vi "Log Data.vi"(8 "error in (no error)":T1 caption="entrée d'erreur (pas d'erreur)", 10 "File d'attente de données":refnum<queue>, 11 "Configuration de l'enregistrement":T2) -> (0 "error out":T1 caption="sortie d'erreur")   [LabVIEW 2018, in "Logging.lvlib"]
doc: "Ce VI utilise la fonction TDMS - Écrire pour écrire des données dans un fichier TDMS."
uses:
  Logging.lvlib
  Logging Configuration.ctl
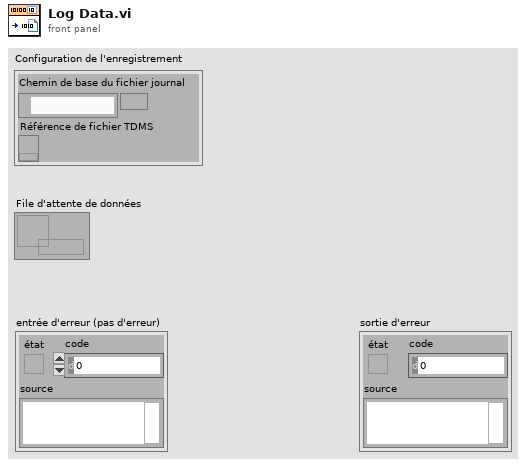
[diagram p1: front panel]
types:
  T1 = cluster{"état":bool, "code":i32, "source":string}
  T2 = typedef "Logging.lvlib/Logging Configuration.ctl" = cluster{"Chemin de base du fichier journal":path, "Référence de fichier TDMS":refnum<k34>}
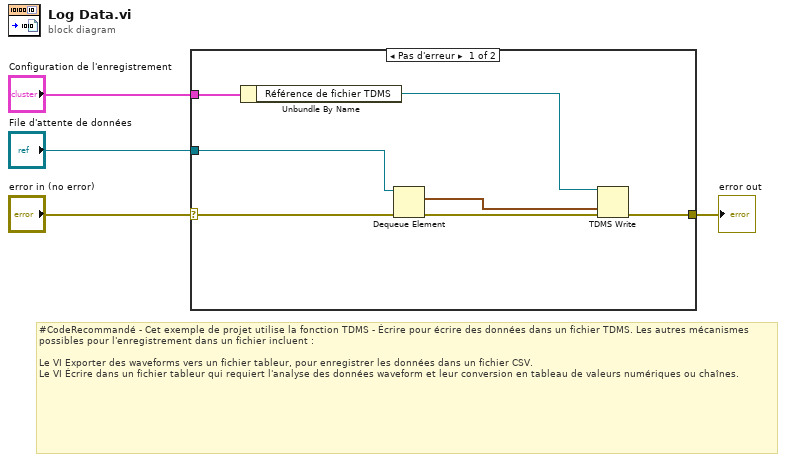
[diagram p0: block diagram]
diagram:
  # "#CodeRecommandé - Cet exemple de projet utilise la fonction TDMS - Écrire pour écrire des données dans un fichier TDMS. Les autres mécanismes possibles pour l'enregistrement dans un fichier incluent :\n\nLe VI Exporter des waveforms vers un fichier tableur, pour enregistrer les données dans un fichier CSV.\nLe VI Écrire dans un fichier tableur qui requiert l'analyse des données waveform et leur conversion en tableau de valeurs numériques ou chaînes."
  n1 = case shown="Pas d'erreur" "error in (no error)" {
    selector: "error in (no error)" -> [w9 w12]
    tunnel: "Configuration de l'enregistrement" -> [w11 _]
    tunnel: "File d'attente de données" -> [w8 _]
    tunnel: [w10 w12] -> w2
    frame No Error {
      n2 = Unbundle By Name(w11) -> ("Référence de fichier TDMS"=w5:refnum<k34>)
      n3 = Dequeue Element(queue=w8, error in (no error)=w9) -> (element=w6:waveform(dbl)[], error out=w7:errorcluster)  [unwired: 1 in, 2 out]
      n4 = TDMS Write(0:w5, 9:w6, 11:w7) -> (15:w10:errorcluster)  [unwired: 3 in, 3 out]
    }
    frame Error {
    }
  }
  "error out" <- w2
